vi "Initialize.vi"(7 "Channel Name":string="Setpoint.ch%d.SP", 8 "error in":errorcluster, 9 "Number of Channels":u32=1, 10 "Instance Name":string="PluginName", 11 "Gradient in":refnum<class "Gradient.lvclass">) -> (0 "error out":errorcluster, 2 "Channel":T1[](array[typedef]), 3 "Gradient out":refnum<class "Gradient.lvclass">)   [LabVIEW 2023, in "Gradient.lvclass"]
uses:
  Gradient.lvclass
  Utilities/Channel.ctl
  Gradient.lvclass/Gradient.ctl
  <vilib>/ADAS Replay HIL/Channels/Tag Wrapper/Polymorphic/Open Consumer Tag (Double).vi
  <vilib>/ADAS Replay HIL/Channels/Tag Wrapper/Polymorphic/Set Default Value (Double).vi
  <vilib>/ADAS Replay HIL/Channels/Tag Wrapper/Polymorphic/Open Consumer Tag (Double).vi/bacb721e-673a-491a-accd-959f2e1f334e.vi
  <vilib>/ADAS Replay HIL/Channels/Tag Wrapper/Polymorphic/Set Default Value (Double).vi/228e99de-6fcf-414d-86fc-dc277c7b351f.vi
  <vilib>/ADAS Replay HIL/Channels/Tag Wrapper/Polymorphic/Open Consumer Tag (Double).vi/bacb721e-673a-491a-accd-959f2e1f334e.vi/c28b0ead-42ad-4072-80a2-aca7f2bd7ce3.vi
  <vilib>/ADAS Replay HIL/Channels/Tag Wrapper/Polymorphic/Set Default Value (Double).vi/228e99de-6fcf-414d-86fc-dc277c7b351f.vi/4bc1c15b-36ab-481f-b8dd-c64075ce723a.vi
  <vilib>/ADAS Replay HIL/AdasHilServices/AdasHilServices Fill In Error Info Ex.vi
  <vilib>/ADAS Replay HIL/Channels/Tag Wrapper/Tag Wrapper.lvlib
  Utilities/Utilities.lvlib
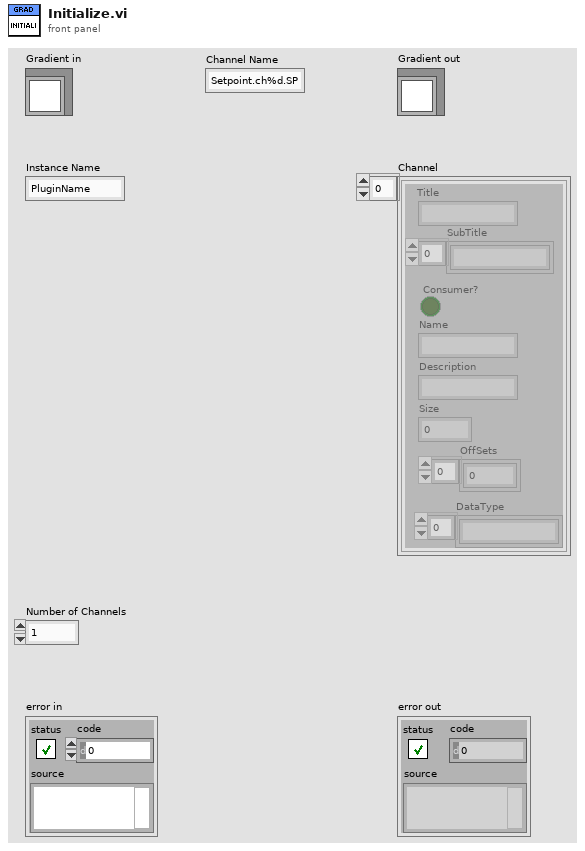
[diagram p1: front panel]
types:
  T1 = typedef "Utilities.lvlib/Channel.ctl" = cluster{"Title":string, "SubTitle":string[], "Consumer?":bool, "Name":string, "Description":string, "Size":i32, "OffSets":i32[], "DataType":string[]}
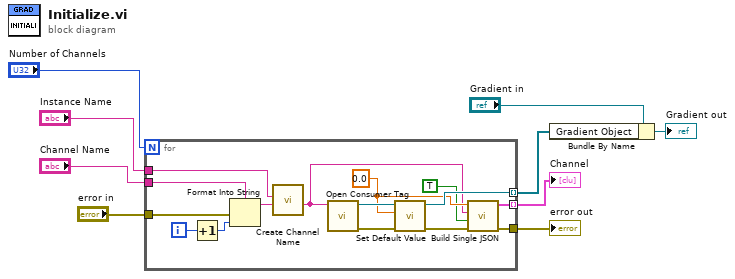
[diagram p0: block diagram]
diagram:
  n1 = for {
    N: "Number of Channels" -> [_]
    tunnel: [w14] -> w2
    tunnel: "Channel Name" -> [w21]
    tunnel: "Instance Name" -> [w20]
    tunnel: "error in" -> [w22]
    tunnel: [w17] -> w5 mode=indexing
    tunnel: [w10] -> w1 mode=indexing
    i -> [w24]
    w13 = 0.0 ("Default Value")
    n2 = Increment(x=w24) -> (x+1=w23:i32)
    n3 = Format Into String(format string=w21, error in=w22, w23) -> (resulting string=w19:string)  [unwired: 1 in, 1 out]
    n4 = call "Create Channel Name.vi"("Channel Name"=w19, "Plugin Name"=w20) -> ("Data Channel Name"=w12:string)  [unwired: 8 in, 1 out]
    n5 = call-poly <vilib>:"Open Consumer Tag.vi"("Channel Name"=w12) -> ("error out"=w16:errorcluster, "ADAS HIL Channel"=w18:refnum<k21>)  [unwired: 9 in]
    n6 = call-poly <vilib>:"Set Default Value.vi"("error in"=w16, "Default Value"=w13, "ADAS HIL Channel in"=w18) -> ("error out"=w15:errorcluster, "ADAS HIL Channel out"=w17:refnum<k21>)  [unwired: 7 in]
    n7 = call "Build Single JSON.vi"("error in"=w15, "Consumer?"=TRUE, "ChannelName"=w12, "Single"=w13) -> ("error out"=w14:errorcluster, "Channel"=w10:T1)  [unwired: 6 in]
  }
  "error out" <- w2
  "Channel" <- w1
  n8 = Bundle By Name(cluster="Gradient in", "Gradient Object"=w5) -> (→"Gradient out":refnum<class "Gradient.lvclass">)
